vi "rtout_controlAQuadBOutClock.vi"(7 "Set":bool, 8 "error in":errorcluster, 9 "clock [ns]":i32, 10 "axis in":u8, 11 "connection ID":refnum<k5>) -> (0 "error out":errorcluster, 1 "clock out [ns]":i32, 2 "axis out":i32, 3 "connection ID":refnum<k5>)   [LabVIEW 2016]
doc: "This function retrieves or sets the clock for AQuadB output."
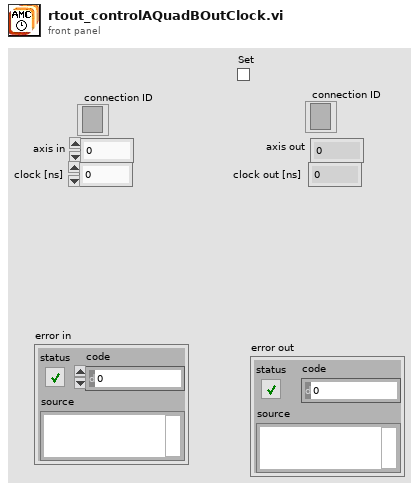
[diagram p1: front panel]
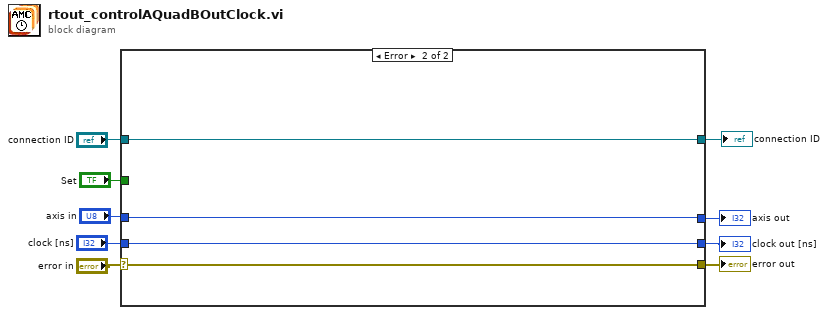
[diagram p0: block diagram]
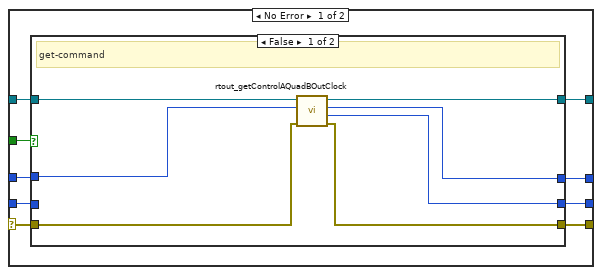
[diagram p2: hidden frame]
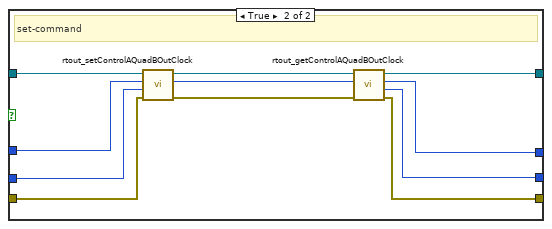
[diagram p3: hidden frame]
diagram:
  n1 = case shown="Error" "error in" {
    selector: "error in" -> [w14 w40]
    tunnel: "axis in" -> [w18 w38]
    tunnel: [w11 w40] -> w8
    tunnel: "clock [ns]" -> [w16 w39]
    tunnel: [w13 w39] -> w3
    tunnel: "Set" -> [w15 _]
    tunnel: [w12 w37] -> w6
    tunnel: "connection ID" -> [w17 w37]
    tunnel: [w10 w38] -> w1
    frame No Error {
      n2 = case shown="False" w15 {
        tunnel: w17 -> [w25 w35]
        tunnel: w18 -> [w22 w27]
        tunnel: w16 -> [_ w28]
        tunnel: w14 -> [w23 w32]
        tunnel: [w20 w29] -> w13
        tunnel: [w24 w33] -> w12
        tunnel: [w21 w31] -> w11
        tunnel: [w19 w30] -> w10
        frame False {
          # "get-command"
          n3 = call "rtout_getControlAQuadBOutClock.vi"("error in"=w23, "axis"=w22, "connection ID"=w25) -> ("error out"=w21:errorcluster, "clock_in_ns"=w20:i32, "axis_out"=w19:i32, "connection ID"=w24:refnum<k5>)  [unwired: 5 in]
        }
        frame True {
          # "set-command"
          n4 = call "rtout_setControlAQuadBOutClock.vi"("error in"=w32, "clock"=w28, "axis"=w27, "connection ID"=w35) -> ("error out"=w36:errorcluster, "axis_out"=w26:i32, "connection ID"=w34:refnum<k5>)  [unwired: 5 in]
          n5 = call "rtout_getControlAQuadBOutClock.vi"("error in"=w36, "axis"=w26, "connection ID"=w34) -> ("error out"=w31:errorcluster, "clock_in_ns"=w29:i32, "axis_out"=w30:i32, "connection ID"=w33:refnum<k5>)  [unwired: 5 in]
        }
      }
    }
    frame Error {
    }
  }
  "error out" <- w8
  "axis out" <- w1
  "clock out [ns]" <- w3
  "connection ID" <- w6
